vi "MVE Project Browse.vi"(10 "Item Path":string, 11 "InitPath":string) -> (3 "outPath":string)   [LabVIEW 2016]
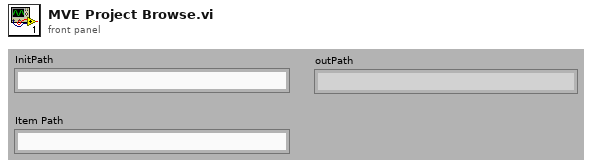
[diagram p1: front panel]
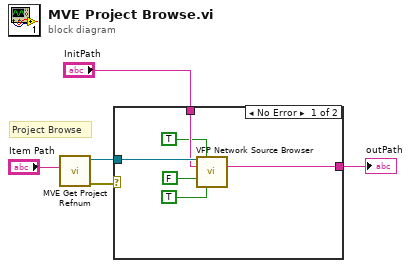
[diagram p0: block diagram]
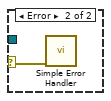
[diagram p2: hidden frame]
diagram:
  # "Project Browse"
  n1 = call <resource>:"MVE Get Project Refnum.vi"("Full Path"="Item Path") -> ("error out"=w1:errorcluster, "Project Refnum"=w2:refnum<vi>)  [unwired: 9 in]
  n2 = case shown="No Error" w1 {
    selector: w1 -> [_ w12]
    tunnel: [w11 _] -> w5
    tunnel: w2 -> [w10 _]
    tunnel: "InitPath" -> [w9 _]
    frame No Error {
      n3 = call <resource>:"VFP Network Source Browser.vi"("Project Refnum"=w10, "Include IO Vars? (F)"=TRUE ("IO Vars only?"), "InitPath"=w9, "MatchChkBox(T)?"=FALSE, "Project Only?"=TRUE) -> ("outPath"=w11:string)  [unwired: 5 in, 5 out]
    }
    frame Error {
      n4 = call <vilib>:"Simple Error Handler.vi"("error in (no error)"=w12) -> ()  [unwired: 4 in, 5 out]
    }
  }
  "outPath" <- w5
